vi "Query Status Questionable Event.vi"(8 "error in":errorcluster, 11 "VISA resource name":refnum<visa-resource-name>) -> (0 "error out":errorcluster, 1 "Value":i32, 3 "VISA resource name out":refnum<visa-resource-name>)   [LabVIEW 2015, in "IT-M7700.lvlib"]
doc: "This command can be used to read the value of the query event register. This is a read-only register that can store the locking event information through the PTR/NTR filter. After this command is executed, the value of the query event register is cleared."
uses:
  <instrlib>/IT-M7700/IT-M7700.lvlib
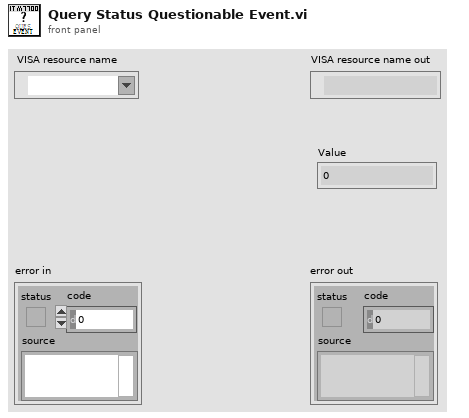
[diagram p1: front panel]
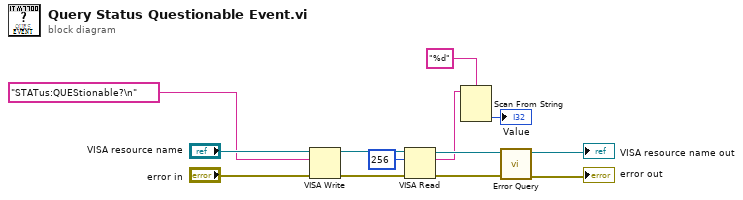
[diagram p0: block diagram]
diagram:
  n1 = VISA Write(VISA resource name="VISA resource name", write buffer="STATus:QUEStionable?\n", error in (no error)="error in") -> (VISA resource name out=w8:refnum<visa-resource-name>, error out=w7:errorcluster)  [unwired: 1 out]
  n2 = VISA Read(VISA resource name=w8, byte count=u32 256 ("字节总数"), error in (no error)=w7) -> (VISA resource name out=w5:refnum<visa-resource-name>, read buffer=w3:string, error out=w6:errorcluster)  [unwired: 1 out]
  n3 = Scan From String(format string="%d" ("格式字符串"), input string=w3) -> (output 1=→"Value":i32)  [unwired: 3 in, 3 out]
  n4 = call <instrlib>:"Error Query.vi"("error in"=w6, "VISA resource name"=w5) -> ("error out"=→"error out":errorcluster, "VISA resource name out"=→"VISA resource name out":refnum<visa-resource-name>)  [unwired: 6 in, 2 out]
